vi "IMAQdx Enumerate Cameras.vi"(8 "error in":errorcluster, 11 "Connected Only? (Yes)":bool=TRUE) -> (0 "error out":errorcluster, 3 "Camera Information Array":T1(array[cluster]) {"BusType" format="%x"; "SerialNumberLow" format="%.0x"; "SerialNumberHigh" format="%.0x"})   [LabVIEW 2020, in "NI_Vision_Acquisition_Software.lvlib"]
doc: "Returns a list of all cameras on the host computer."
uses:
  NI_Vision_Acquisition_Software.lvlib
  niimaqdx.dll
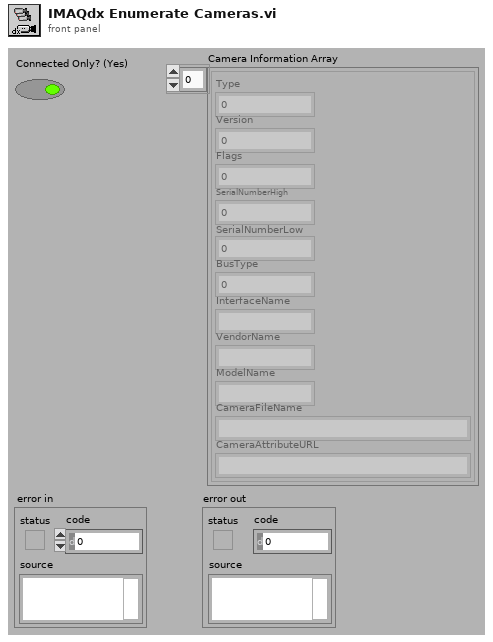
[diagram p1: front panel]
types:
  T1 = cluster{"Type":u32, "Version":u32, "Flags":u32, "SerialNumberHigh":u32, "SerialNumberLow":u32, "BusType":u32, "InterfaceName":string, "VendorName":string, "ModelName":string, "CameraFileName":string, "CameraAttributeURL":string}[]
  T2 = cluster{"Type":u32, "Version":u32, "Flags":u32, "SerialNumberHi":u32, "SerialNumberLo":u32, "BusType":u32, "InterfaceName":string, "VendorName":string, "ModelName":string, "CameraFileName":string, "CameraAttributeURL":string}[]
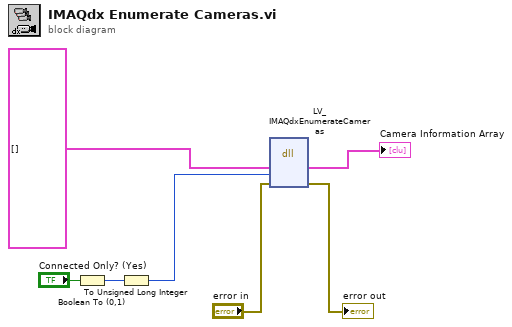
[diagram p0: block diagram]
diagram:
  n1 = Boolean To (0,1)(Boolean="Connected Only? (Yes)") -> (0, 1=w4:i16)
  n2 = To Unsigned Long Integer(number=w4) -> (unsigned 32bit integer=w3:u32)
  n3 = dll-call lib="niimaqdx.dll" fn="LV_IMAQdxEnumerateCameras"("Camera Information Array"=T2 [], "connectedOnly"=w3, "error in"="error in") -> ("Camera Information Array"=→"Camera Information Array":T2, "error in"=→"error out":errorcluster)  [unwired: 5 in, 2 out]
